vi "HeaderStrings.vi"(8 "Units":dbl, 10 "ASCIIstringIn":string, 11 "Type":T1(ring)) -> (3 "ASCIIstringOut":string)   [LabVIEW 2012]
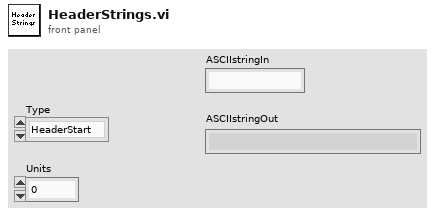
[diagram p1: front panel]
types:
  T1 = enum16{"HeaderStart", "HeaderEnd", "Binary", "Units"}
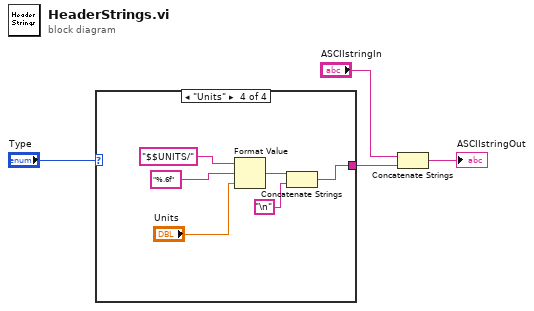
[diagram p0: block diagram]
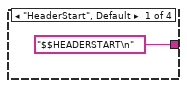
[diagram p2: hidden frame]
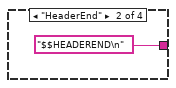
[diagram p3: hidden frame]
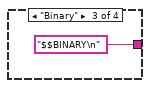
[diagram p4: hidden frame]
diagram:
  n1 = case shown="\"Units\"" "Type" {
    tunnel: ["$$HEADERSTART\n" ("String") "$$HEADEREND\n" ("String") "$$BINARY\n" ("String") w9] -> w3
    frame "HeaderStart", Default {
    }
    frame "HeaderEnd" {
    }
    frame "Binary" {
    }
    frame "Units" {
      n2 = Format Value(string ("")="$$UNITS/" ("string"), format string="%.6f", value (0)="Units") -> (output string=w10:string)
      n3 = Concatenate Strings(w10, "\n") -> (w9:string)
    }
  }
  n4 = Concatenate Strings("ASCIIstringIn", w3) -> (→"ASCIIstringOut":string)
